vi "Step Gate Voltage.vi"(0 "Scan Values":T1={"Min Vg (V)"=0.0, "Max Vg (V)"=10.0, "Vm Start (V)"=5.0, "Vm Stop (V)"=9.0, "Steps/Sec"=100.0, "Vm Rate (Hz)"=100.0, "Wavelength Start (nm)"=450.0, "Wavelength Stop (nm)"=850.0, "Wavelength Step (nm)"=2.0, "Vsd (V)"=0.1, "Vg Step Size"=0.01, "Vsd Ramp Time (secs)"=0.1} {"Vsd Ramp Time (secs)" min=-10.0 max=10.0; "Vg Step Size" min=0.0 max=0.5; "Vsd (V)" min=-10.0 max=10.0; "Wavelength Step (nm)" min=0.0 max=500.0; "Wavelength Stop (nm)" min=16.0 max=2500.0; "Wavelength Start (nm)" min=15.0 max=2499.0; "Steps/Sec" min=1.0 max=1000.0; "Vm Stop (V)" min=-10.0 max=10.0; "Vm Start (V)" min=-10.0 max=10.0; "Max Vg (V)" min=-9.9 max=10.0; "Min Vg (V)" min=-10.0 max=9.9}, 1 "Vg Value (V)":dbl, 2 "Direction":bool=TRUE) -> (3 "New Vg Value (V)":dbl, 4 "New Direction":bool, 5 "High/Low":u16, 6 "Out of Range":bool)   [LabVIEW 2009]
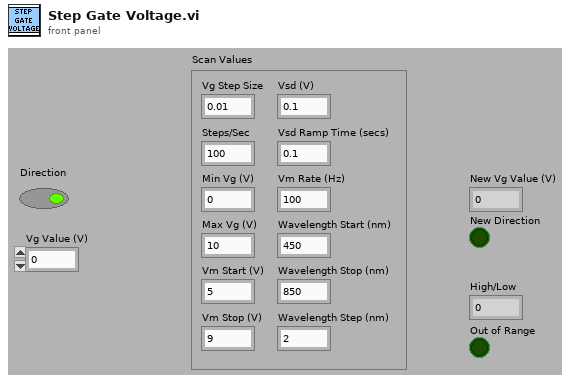
[diagram p1: front panel]
types:
  T1 = cluster{"Min Vg (V)":dbl, "Max Vg (V)":dbl, "Vm Start (V)":dbl, "Vm Stop (V)":dbl, "Steps/Sec":dbl, "Vm Rate (Hz)":dbl, "Wavelength Start (nm)":dbl, "Wavelength Stop (nm)":dbl, "Wavelength Step (nm)":dbl, "Vsd (V)":dbl, "Vg Step Size":dbl, "Vsd Ramp Time (secs)":dbl}
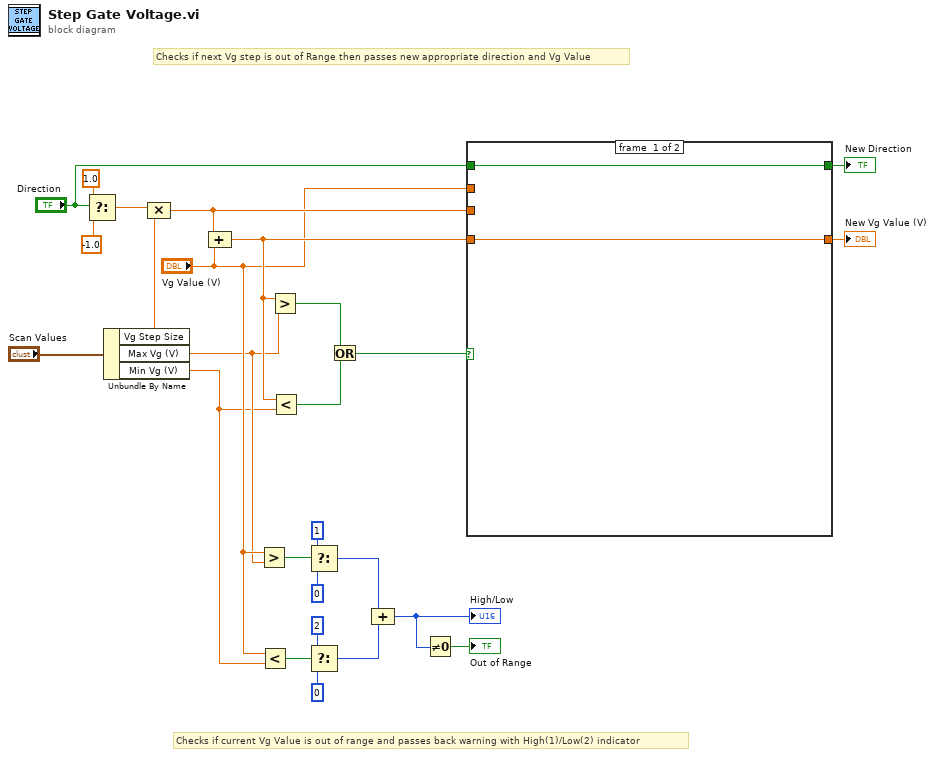
[diagram p0: block diagram]
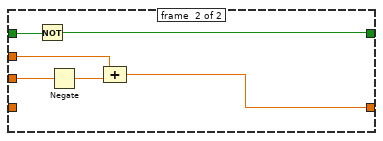
[diagram p2: hidden frame]
diagram:
  # "Checks if current Vg Value is out of range and passes back warning with High(1)/Low(2) indicator"
  # "Checks if next Vg step is out of Range then passes new appropriate direction and Vg Value"
  n1 = Select(t=1.0, s="Direction", f=-1.0) -> (s? t:f=w24:dbl)
  n2 = Unbundle By Name("Scan Values") -> ("Vg Step Size"=w21:dbl, "Max Vg (V)"=w16:dbl, "Min Vg (V)"=w15:dbl)
  n3 = Compound Arithmetic op=MULTIPLY(w24, w21) -> (w18:dbl)
  n4 = Compound Arithmetic op=ADD(w18, "Vg Value (V)") -> (w22:dbl)
  n5 = Greater?(x="Vg Value (V)", y=w16) -> (0:w10:bool)
  n6 = Less?(x="Vg Value (V)", y=w15) -> (x < y?=w9:bool)
  n7 = Greater?(x=w22, y=w16) -> (0:w4:bool)
  n8 = Less?(x=w22, y=w15) -> (x < y?=w3:bool)
  n9 = Select(t=u16 1, s=w10, f=u16 0) -> (s? t:f=w8:u16)
  n10 = Select(t=u16 2, s=w9, f=u16 0) -> (s? t:f=w7:u16)
  n11 = Or(x=w4, y=w3) -> (x .or. y?=w2:bool)
  n12 = Compound Arithmetic op=ADD(w8, w7) -> (w6:u16)
  "High/Low" <- w6
  n13 = Not Equal To 0?(x=w6) -> (x != 0?=→"Out of Range":bool)
  n14 = case shown="True" w2 {
    tunnel: "Direction" -> [w28 w33]
    tunnel: w22 -> [w27 _]
    tunnel: [w28 w32] -> w19
    tunnel: [w27 w29] -> w20
    tunnel: "Vg Value (V)" -> [_ w30]
    tunnel: w18 -> [_ w34]
    frame #0 {
    }
    frame #1 {
      n15 = Not(x=w33) -> (.not. x?=w32:bool)
      n16 = Negate(x=w34) -> (-x=w31:dbl)
      n17 = Compound Arithmetic op=ADD(w30, w31) -> (w29:dbl)
    }
  }
  "New Vg Value (V)" <- w20
  "New Direction" <- w19
